vi "SetUp.vi"(8 "error in (no error)":errorcluster, 11 "Prueba08 in":refnum<class "Prueba32.lvclass">) -> (0 "error out":errorcluster, 3 "Prueba08 out":refnum<class "Prueba32.lvclass">)   [LabVIEW 2019, in "Prueba32.lvclass"]
uses:
  Prueba32.lvclass
  Prueba32.lvclass/Prueba32.ctl
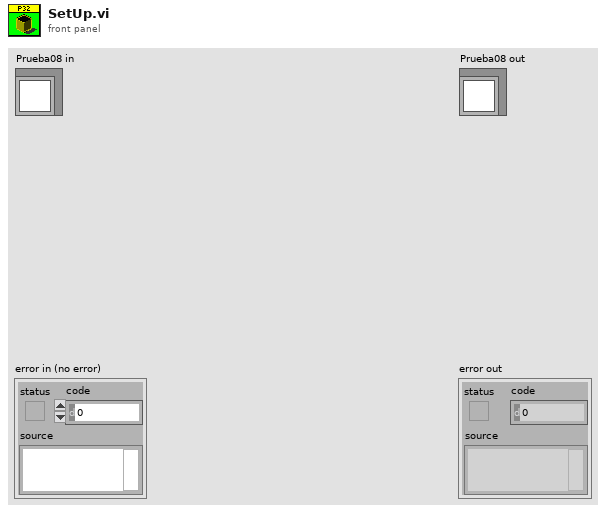
[diagram p1: front panel]
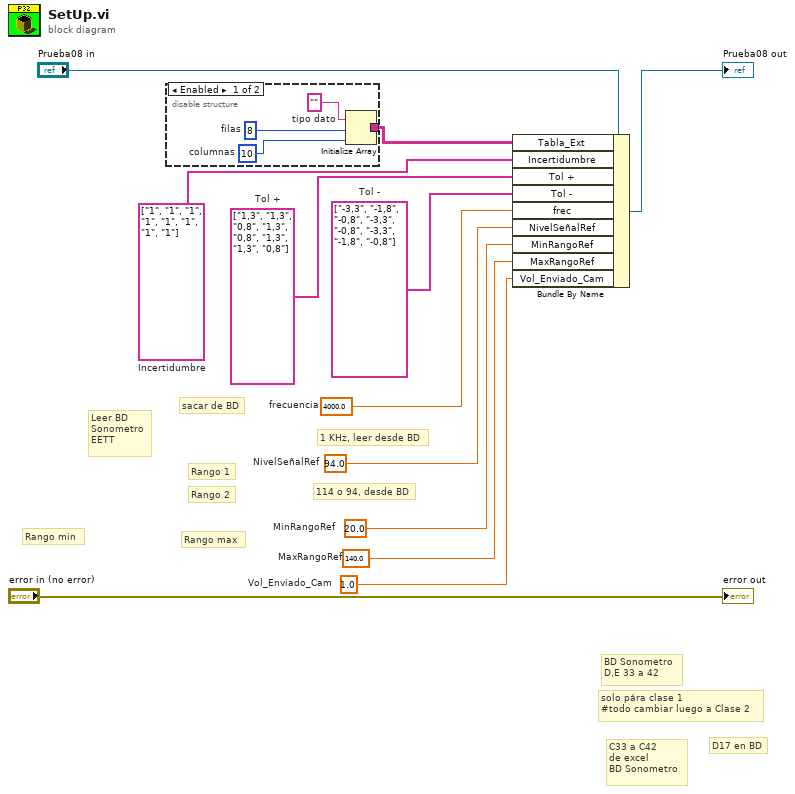
[diagram p0: block diagram]
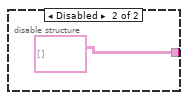
[diagram p2: hidden frame]
diagram:
  w1 = 1.0  # Vol_Enviado_Cam
  w2 = 140.0  # MaxRangoRef
  w3 = 20.0  # MinRangoRef
  w11 = 94.0  # NivelSeñalRef
  w10 = 4000.0  # frecuencia
  w9 = string[] ["1", "1", "1", "1", "1", "1", "1", "1"]  # Incertidumbre
  w8 = string[] ["-3,3", "-1,8", "-0,8", "-3,3", "-0,8", "-3,3", "-1,8", "-0,8"]  # Tol -
  w7 = string[] ["1,3", "1,3", "0,8", "1,3", "0,8", "1,3", "1,3", "0,8"]  # Tol +
  # "114 o 94, desde BD"
  # "1 KHz, leer desde BD"
  # "Rango 2"
  # "Rango 1"
  # "Rango max"
  # "Rango min"
  # "Leer BD\nSonometro\nEETT"
  # "sacar de BD"
  # "D17 en BD"
  # "BD Sonometro\nD,E 33 a 42"
  # "solo pára clase 1\n#todo cambiar luego a Clase 2"
  # "C33 a C42\nde excel\nBD Sonometro"
  n1 = disable-structure shown="Enabled" {
    disable-tunnel: [w13 string[][] []] -> w6
    frame Enabled {
      w15 = 10  # columnas
      w14 = 8  # filas
      w16 = ""  # tipo dato
      n2 = Initialize Array(w16, w14, w15) -> (w13:string[][])
    }
    frame Disabled {
    }
  }
  n3 = Bundle By Name(cluster="Prueba08 in", "Tabla_Ext"=w6, "Incertidumbre"=w9, "Tol +"=w7, "Tol -"=w8, "frec"=w10, "NivelSeñalRef"=w11, "MinRangoRef"=w3, "MaxRangoRef"=w2, "Vol_Enviado_Cam"=w1) -> (→"Prueba08 out":refnum<class "Prueba32.lvclass">)
  "error out" <- "error in (no error)"
